vi "Add Pulse Recorders.vi"(8 "error in (no error)":errorcluster, 9 "Auto launch":bool=TRUE, 10 "String":string, 11 "LabActor in":refnum<class "LabActor.lvclass">) -> (0 "error out":errorcluster, 1 "Actor names out":string[](array[string]), 2 "Recorders out":refnum<class "Pulse Recorder Actor.lvclass">[](array[class]), 3 "LabActor out":refnum<class "LabActor.lvclass">, 4 "Type IDs":i32[](array[numeric]), 5 "Add to monitor":bool[](array[boolean]))   [LabVIEW 2024, in "LabActor.lvclass"]
uses:
  LabActor.lvclass
  Pulse Recorders/Pulse Recorder Actor/Pulse Recorder Actor.lvclass
  NHMFL_Core/Libraries/Instruments/Micron Optics/Micron sm Digitizer/Micron sm Digitizer.lvclass
  Recorders/Micron Optics/Micron Optics Recorder.lvclass
  Recorders/RP I-V/RP I-V.lvclass
  Recorders/RP Delayed/RP Modulated.lvclass
  Recorders/RP Level/RP Level.lvclass
  Recorders/NI-Scope Lock-in/NI-Scope Lock-in.lvclass
  Pulse Recorders/Lockin Digitizer/Lockin Digitizer.lvclass
  Recorders/Waveform Generator/Waveform Generator.lvclass
  NHMFL_Core/Libraries/Red Pitaya/Red Pitaya Digitizer/Red Pitaya Digitizer.lvclass
  NHMFL_Core/Libraries/Instruments/Pulse Driver/Pulse Driver.lvclass
  LabActor.lvclass/LabActor.ctl
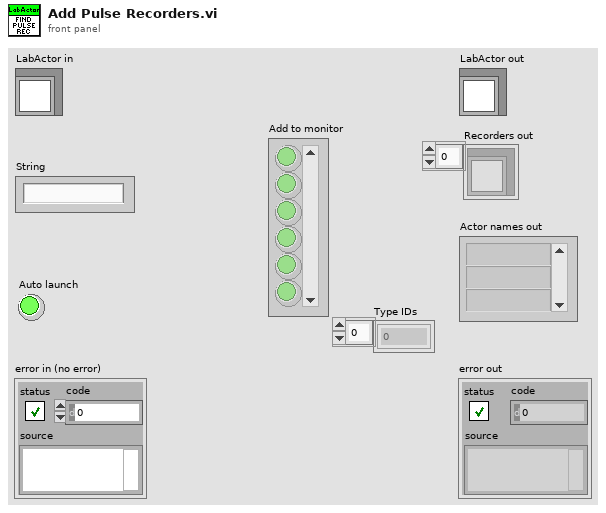
[diagram p1: front panel]
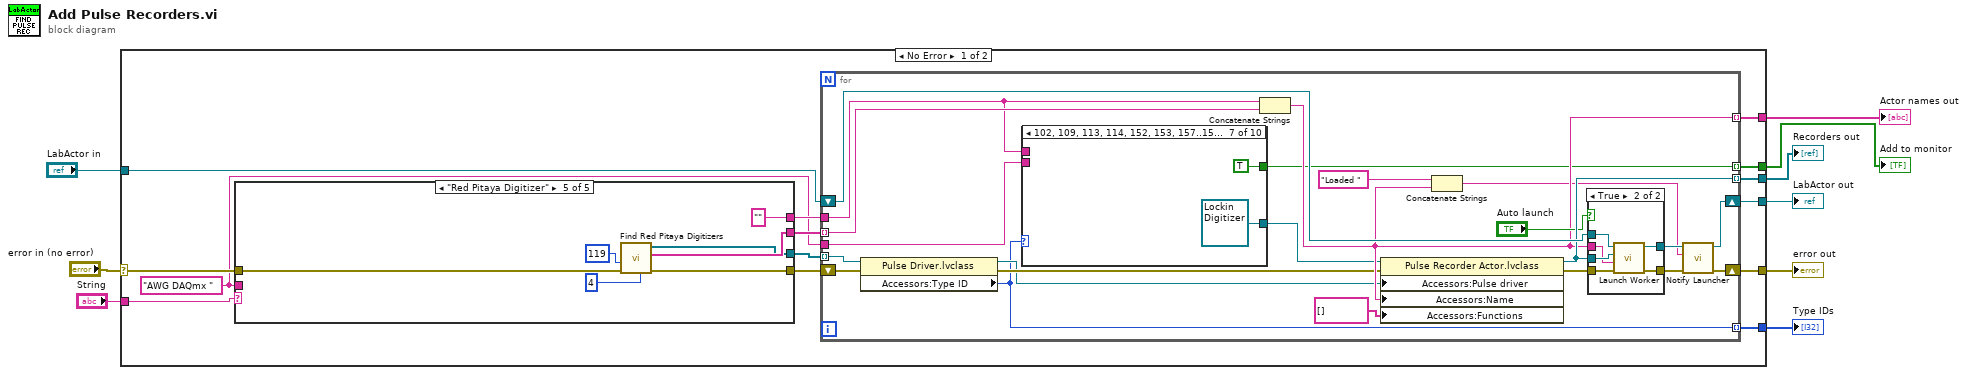
[diagram p0: block diagram]
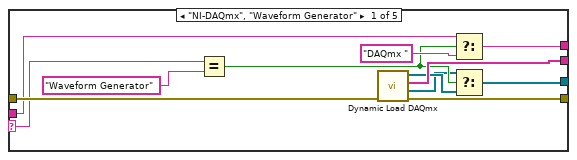
[diagram p2: hidden frame]
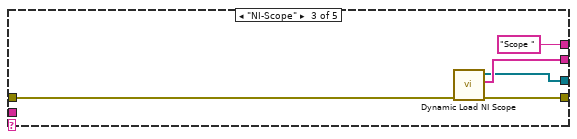
[diagram p4: hidden frame]
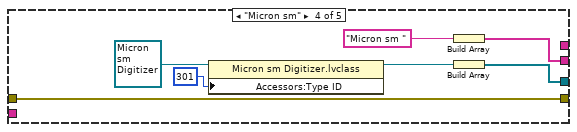
[diagram p5: hidden frame]
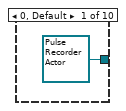
[diagram p6: hidden frame]
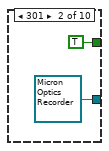
[diagram p7: hidden frame]
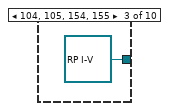
[diagram p8: hidden frame]
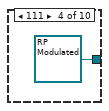
[diagram p9: hidden frame]
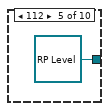
[diagram p10: hidden frame]
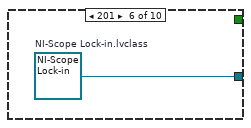
[diagram p11: hidden frame]
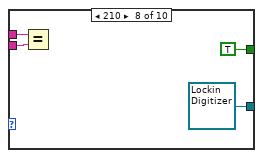
[diagram p12: hidden frame]
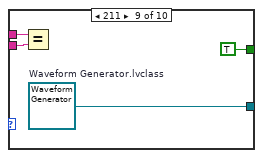
[diagram p13: hidden frame]
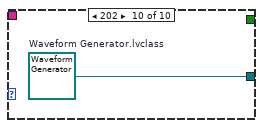
[diagram p14: hidden frame]
diagram:
  n1 = case shown="No Error" "error in (no error)" {
    selector: "error in (no error)" -> [w23 w105]
    tunnel: [w19 w105] -> w8
    tunnel: [w15 w104] -> w6
    tunnel: "LabActor in" -> [w16 w104]
    tunnel: [w18 _] -> w5
    tunnel: [w17 _] -> w4
    tunnel: "String" -> [w14 _]
    tunnel: [w12 _] -> w2
    tunnel: [w11 _] -> w1
    frame No Error {
      w10 = "AWG DAQmx "
      n2 = case shown="\"Red Pitaya Digitizer\"" w14 {
        selector: w14 -> [w32 _ _ _ _]
        tunnel: w23 -> [w35 w36 w41 w48 w55]
        tunnel: [w26 _ w38 w47 w52] -> w22
        tunnel: [w34 w36 w40 w48 w51] -> w21
        tunnel: [w33 _ w39 w43 w54] -> w20
        tunnel: [w29 _ "Scope " _ ""] -> w13
        tunnel: w10 -> [w28 _ _ _ _]
        frame "NI-DAQmx", "Waveform Generator" {
          n3 = Equal?(x=w32, y="Waveform Generator") -> (x = y?=w27:bool)
          n4 = call "Dynamic Load DAQmx.vi"("Error In"=w35) -> ("Error Out"=w34:errorcluster, "Synthesizers Out"=w24:refnum<class "Pulse Driver.lvclass">[], "Device names"=w33:string[], "Digitizers out"=w25:refnum<class "Pulse Driver.lvclass">[])  [unwired: 7 in]
          n5 = Select(t=w28, s=w27, f="DAQmx ") -> (s? t:f=w29:string)
          n6 = Select(t=w24, s=w27, f=w25) -> (s? t:f=w26:refnum<class "Pulse Driver.lvclass">[])
        }
        frame "NONE", Default {
        }
        frame "NI-Scope" {
          n7 = call "Dynamic Load NI Scope.vi"("Error In"=w41) -> ("Error Out"=w40:errorcluster, "Device names"=w39:string[], "Digitizers out"=w38:refnum<class "Pulse Driver.lvclass">[])  [unwired: 8 in]
        }
        frame "Micron sm" {
          n8 = property class="Micron sm Digitizer.lvclass"(reference=refnum<class "Micron sm Digitizer.lvclass"> refnum ("Micron sm Digitizer.lvclass"), "Accessors:Type ID"=301 ("Type ID")) -> (reference out=w46:refnum<class "Micron sm Digitizer.lvclass">)  [unwired: 1 in, 1 out]
          n9 = Build Array("Micron sm ") -> (w43:string[])
          n10 = Build Array(w46) -> (w47:refnum<class "Micron sm Digitizer.lvclass">[])
        }
        frame "Red Pitaya Digitizer" {
          n11 = call "Find Red Pitaya Digitizers.vi"("Find linked modules"=4 ("Find initiator-follower couples"), "Error In"=w55, "End address for stand-alone"=119 ("End address")) -> ("Error Out"=w51:errorcluster, "Device names"=w54:string[], "Digitizers out"=w52:refnum<class "Red Pitaya Digitizer.lvclass">[])  [unwired: 5 in, 1 out]
        }
      }
      n12 = for {
        tunnel: w22 -> [w63] mode=indexing
        shift-right: [w69] -> w19
        shift-left: w21 -> [w77]
        tunnel: w20 -> [w60] mode=indexing
        tunnel: [w75] -> w18 mode=indexing
        tunnel: [w67] -> w17 mode=indexing
        shift-right: [w71] -> w15
        shift-left: w16 -> [w76]
        tunnel: w13 -> [w57]
        tunnel: [w59] -> w12 mode=indexing
        tunnel: [w58] -> w11 mode=indexing
        tunnel: w10 -> [w56]
        n13 = property class="Pulse Driver.lvclass"(reference=w63, error in=w77) -> (reference out=w62:refnum<class "Pulse Driver.lvclass">, error out=w64:errorcluster, "Accessors:Type ID"=w59:i32)
        n14 = case shown="102, 109, 113, 114, 152, 153, 157..159, 164, 169" w59 {
          tunnel: [refnum<class "Pulse Recorder Actor.lvclass"> refnum ("Pulse Recorder.lvclass") refnum<class "Micron Optics Recorder.lvclass"> refnum ("Pulse Recorder.lvclass") refnum<class "RP I-V.lvclass"> refnum ("RP I-V.lvclass") refnum<class "RP Modulated.lvclass"> refnum ("RP Delayed.lvclass") refnum<class "RP Level.lvclass"> refnum ("RP Level.lvclass") w84 refnum<class "Lockin Digitizer.lvclass"> refnum ("Lockin Digitizer.lvclass") refnum<class "Lockin Digitizer.lvclass"> refnum ("Lockin Digitizer.lvclass") w91 w95] -> w61
          tunnel: [_ TRUE _ _ _ _ TRUE TRUE TRUE _] -> w58
          tunnel: w57 -> [_ _ _ _ _ _ _ w89 w93 _]
          tunnel: w56 -> [_ _ _ _ _ _ _ w88 w92 _]
          frame 0, Default {
          }
          frame 301 {
          }
          frame 104, 105, 154, 155 {
          }
          frame 111 {
          }
          frame 112 {
          }
          frame 201 {
            w84 = refnum<class "NI-Scope Lock-in.lvclass"> refnum  # NI-Scope Lock-in.lvclass
          }
          frame 102, 109, 113, 114, 152, 153, 157..159, 164, 169 {
          }
          frame 210 {
            n15 = Equal?(x=w89, y=w88) -> ()  [unwired: 1 out]
          }
          frame 211 {
            w91 = refnum<class "Waveform Generator.lvclass"> refnum  # Waveform Generator.lvclass
            n16 = Equal?(x=w93, y=w92) -> ()  [unwired: 1 out]
          }
          frame 202 {
            w95 = refnum<class "Waveform Generator.lvclass"> refnum  # Waveform Generator.lvclass
          }
        }
        n17 = Concatenate Strings(w57, w60) -> (w67:string)
        n18 = property class="Pulse Recorder Actor.lvclass"(reference=w61, error in=w64, "Accessors:Pulse driver"=w62, "Accessors:Name"=w67, "Accessors:Functions"=string[] [] ("Functions")) -> (reference out=w75:refnum<class "Pulse Recorder Actor.lvclass">, error out=w74:errorcluster)
        n19 = Concatenate Strings("Loaded " ("string"), w67) -> (w66:string)
        n20 = case shown="True" "Auto launch" {
          tunnel: w76 -> [w97 w103]
          tunnel: w75 -> [_ w102]
          tunnel: [w97 w101] -> w72
          tunnel: w74 -> [w96 w100]
          tunnel: [w96 w99] -> w70
          tunnel: w67 -> [_ w98]
          frame False {
          }
          frame True {
            n21 = call-dynamic "Launch Worker.vi"("error in (no error)"=w100, "Name"=w98, "Subordinate Object"=w102, "Application Controller in"=w103) -> ("error out"=w99:errorcluster, "Application Controller out"=w101:refnum<class "LabActor.lvclass">)  [unwired: 5 in, 1 out]
          }
        }
        n22 = call-dynamic "Notify Launcher.vi"("error in (no error)"=w70, "Notification"=w66, "Application Controller in"=w72) -> ("error out"=w69:errorcluster, "Application Controller out"=w71:refnum<class "LabActor.lvclass">)  [unwired: 7 in]
      }
    }
    frame Error {
    }
  }
  "error out" <- w8
  "LabActor out" <- w6
  "Recorders out" <- w5
  "Actor names out" <- w4
  "Type IDs" <- w2
  "Add to monitor" <- w1
